vi "Get Knock Cylinders - Multi FPGA.vi"(7 "Max angle":dbl, 8 "error in (no error)":errorcluster, 10 "Knock Sensor":string, 11 "Item Ref in":T1 format="%.0x") -> (0 "error out":errorcluster, 1 "cylinder item refs":T1[](array[typedef]) format="%.0x", 2 "cylinders":T2[](array[typedef]), 3 "Item Ref out":T1 format="%.0x", 5 "not present indexes":i32[](array[numeric]))   [LabVIEW 2015, in "Engine Simulation Toolkit System Explorer.lvlib"]
uses:
  Engine Simulation Toolkit System Explorer.lvlib
  Knock Cylinder.ctl
  <vilib>/NI Veristand/Custom Device API/Custom Device Item Ref.ctl
  Shared/Properties.vi
  Shared/Constants and GUIDs.vi
  <vilib>/NI Veristand/Custom Device Tools/Custom Device Utility Library/NI VeriStand - Search for All Items by GUID.vi
  <vilib>/NI Veristand/Custom Device API/Get Item Property (String).vi
  Shared/Engine Simulation Toolkit Shared.lvlib
  <vilib>/NI Veristand/Custom Device API/Custom Device API.lvlib
  <vilib>/NI Veristand/Custom Device Tools/Custom Device Utility Library/Custom Device Utility Library.lvlib
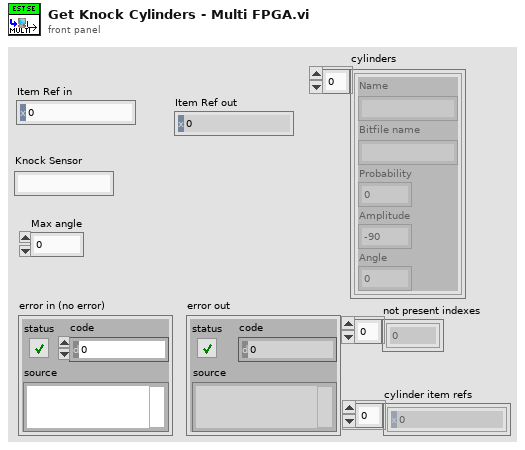
[diagram p1: front panel]
types:
  T1 = typedef "Custom Device API.lvlib/Custom Device Item Ref.ctl" = u64
  T2 = typedef "Engine Simulation Toolkit System Explorer.lvlib/Knock Cylinder.ctl" = cluster{"Name":string, "Bitfile name":string, "Probability":dbl, "Amplitude":dbl, "Angle":dbl}
  T3 = typedef "Engine Simulation Toolkit Shared.lvlib/Channel.ctl" = cluster{"Name":string, "Units":string, "Default":dbl, "Description":string, "Scalable":bool}
  T4 = typedef "Custom Device API.lvlib/Custom Device Channel.ctl" = cluster{"Type":T5, "Units":string, "Default Value":dbl, "Faultable":bool, "Scalable":bool}
  T5 = typedef "Custom Device API.lvlib/Custom Device Channel Type.ctl" = enum16{"Input", "Output"}
  T6 = typedef "Custom Device API.lvlib/Custom Device Item Info.ctl" = cluster{"Name":string, "Is Channel":bool, "GUID":string, "Is Waveform":bool}
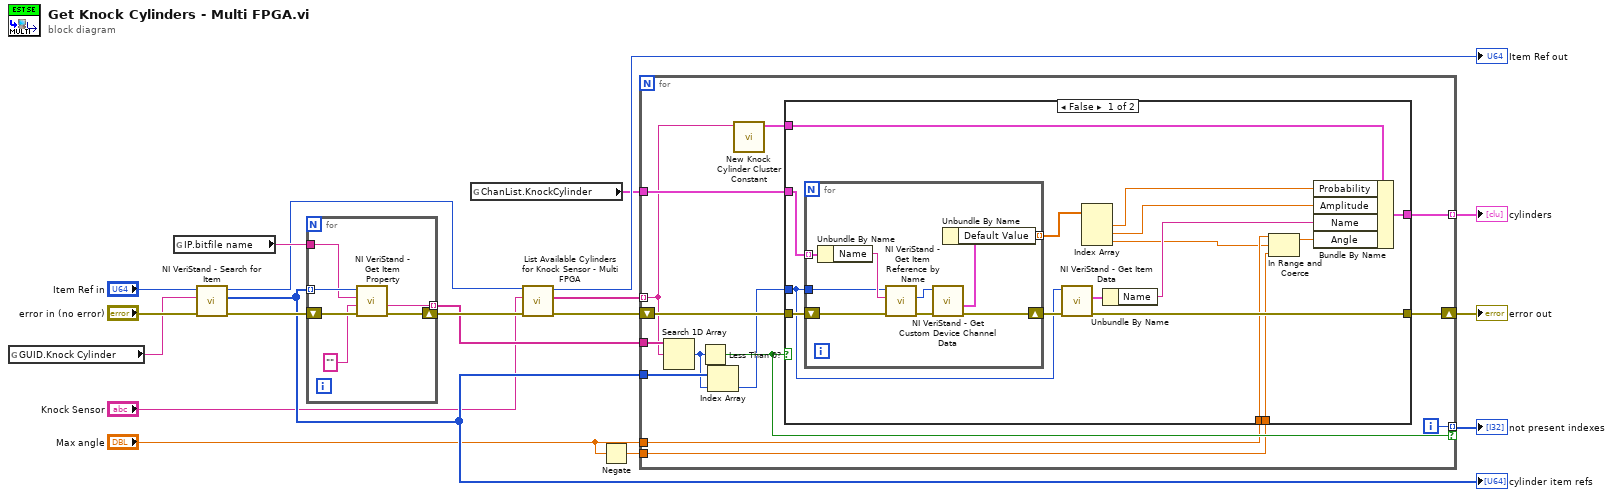
[diagram p0: block diagram]
diagram:
  n1 = global read "Constants and GUIDs.vi" "GUID.Knock Cylinder"() -> (w5:string)
  n2 = global read "Properties.vi" "IP.bitfile name"() -> (w11:string)
  n3 = call-poly <vilib>:"NI VeriStand - Search for Item.vi"("error in"="error in (no error)", "Item GUID"=w5, "Section Ref in"="Item Ref in") -> ("error out"=w12:errorcluster, "Item Refs"=w7:T1[], "Section Ref out"=w10:T1)  [unwired: 5 in, 1 out]
  "cylinder item refs" <- w7
  n4 = for {
    shift-right: [w22] -> w9
    shift-left: w12 -> [w25]
    tunnel: w7 -> [w24] mode=indexing
    tunnel: w11 -> [w23]
    tunnel: [w20] -> w8 mode=indexing
    n5 = call-poly <vilib>:"NI VeriStand - Get Item Property.vi"("error in (no error)"=w25, "Default Value"="", "Property Name"=w23, "Item Ref in"=w24) -> ("error out"=w22:errorcluster, "Value"=w20:string)  [unwired: 4 in, 2 out]
  }
  n6 = global read "Constants and GUIDs.vi" "ChanList.KnockCylinder"() -> (w3:T3[])
  n7 = call "List Available Cylinders for Knock Sensor - Multi FPGA.vi"("error in (no error)"=w9, "Timing measurement"="Knock Sensor", "Item Ref in"=w10) -> ("error out"=w17:errorcluster, "cylinders available"=w16:string[], "Item Ref out"=→"Item Ref out":T1)  [unwired: 6 in]
  n8 = Negate(x="Max angle") -> (-x=w1:dbl)
  n9 = for {
    tunnel: [w28] -> w19 mode=indexing
    shift-right: [w39] -> w14
    shift-left: w17 -> [w37]
    tunnel: w16 -> [w29] mode=indexing
    tunnel: [w38] -> w13 mode=indexing if=w35
    tunnel: w8 -> [w36]
    tunnel: w7 -> [w34]
    tunnel: w3 -> [w31]
    tunnel: "Max angle" -> [w27]
    tunnel: w1 -> [w26]
    i -> [w38]
    n10 = Search 1D Array(1D array=w36, element=w29) -> (index of element=w33:i32)  [unwired: 1 in]
    n11 = Less Than 0?(x=w33) -> (x < 0?=w35:bool)
    n12 = Index Array(array=w34, index=w33) -> (element=w32:T1)
    n13 = call "New Knock Cylinder Cluster Constant.vi"("Bitfile name"=w29) -> ("Knock"=w30:T2)  [unwired: 10 in]
    n14 = case shown="False" w35 {
      tunnel: w37 -> [w50 w66]
      tunnel: w32 -> [w44 _]
      tunnel: [w55 w66] -> w39
      tunnel: w31 -> [w48 _]
      tunnel: w30 -> [w53 w65]
      tunnel: [w51 w65] -> w28
      tunnel: w27 -> [w42 _]
      tunnel: w26 -> [w41 _]
      frame False {
        n15 = for {
          shift-right: [w59] -> w49
          shift-left: w50 -> [w64]
          tunnel: w48 -> [w63] mode=indexing
          tunnel: w44 -> [w61]
          tunnel: [w57] -> w47 mode=indexing
          n16 = Unbundle By Name(w63) -> ("Name"=w62:string)
          n17 = call <vilib>:"NI VeriStand - Get Item Reference by Name.vi"("error in (no error)"=w64, "Item Name"=w62, "Parent Ref in"=w61) -> ("error out"=w60:errorcluster, "Item Ref"=w56:T1)  [unwired: 5 in, 2 out]
          n18 = call <vilib>:"NI VeriStand - Get Custom Device Channel Data.vi"("error in (no error)"=w60, "Channel Ref in"=w56) -> ("error out"=w59:errorcluster, "Channel"=w58:T4)  [unwired: 4 in, 4 out]
          n19 = Unbundle By Name(w58) -> ("Default Value"=w57:dbl)
        }
        n20 = call <vilib>:"NI VeriStand - Get Item Data.vi"("error in (no error)"=w49, "Item Ref in"=w44) -> ("error out"=w55:errorcluster, "Item Info"=w54:T6)  [unwired: 6 in, 2 out]
        n21 = Index Array(array=w47) -> (element #1=w46:dbl, element #2=w45:dbl, element #3=w40:dbl)  [unwired: 3 in]
        n22 = Unbundle By Name(w54) -> ("Name"=w52:string)
        n23 = In Range and Coerce(upper limit=w42, x=w40, lower limit=w41) -> (coerced(x)=w43:dbl)  [unwired: 1 out]
        n24 = Bundle By Name(cluster=w53, "Probability"=w46, "Amplitude"=w45, "Name"=w52, "Angle"=w43) -> (w51:T2)
      }
      frame True {
      }
    }
  }
  "error out" <- w14
  "cylinders" <- w19
  "not present indexes" <- w13
